vi "Tx_Create FIFO Association - Scheduled Labels - Parameters Channels.vi"(8 "error in (no error)":errorcluster, 11 "Input Channel Data []":T5[](array[typedef]) {"Labels Settings"."Label Timestamp Channel Data Reference" format="%.0x"; "Labels Settings"."Label Disable/Trigger Channel Reference" format="%.0x"; "Labels Settings"."Word"."Param Setting"."Item Refs" format="%.0x"; "Labels Settings"."Word"."Param Setting"."Num Bits" min=1 max=32; "Labels Settings"."Word"."Param Setting"."Start Bit" min=8 max=31; "Labels Settings"."Label" format="%.0o"}) -> (0 "error out":errorcluster, 2 "Raw Values":T1, 3 "Map":T4[](array[typedef]) {"Channel Data Reference" format="%.0x"})   [LabVIEW 2019, in "Ballard Arinc-429 Engine.lvlib"]
doc: "This VI creates a static association between NI-VS FIFO Channel Index and Physical Channel, Label Index, Parameter Index for Parameter Channel of a Tx Scheduled Label."
uses:
  Ballard Arinc-429 Engine.lvlib
  Shared/Controls and Global/RT HW Channel.ctl
  Shared/Controls and Global/RT Label Settings.ctl
  Shared/Controls and Global/Label.ctl
  Shared/Controls and Global/transferPeriod.ctl
  Shared/Controls and Global/RT Word Settings.ctl
  Shared/Controls and Global/RT Param Setting.ctl
  Shared/Controls and Global/Start Bit.ctl
  Shared/Controls and Global/Number of Bits.ctl
  <vilib>/NI VeriStand/Custom Device API/Block Data Reference.ctl
  <vilib>/NI VeriStand/Custom Device API/Data Reference.ctl
  <vilib>/NI VeriStand/Custom Device API/Custom Device Item Ref.ctl
  Shared/Controls and Global/TransferType.ctl
  RT Controls/RT Tx Association.ctl
  RT Controls/RT Tx Default Raw Value.ctl
  RT Controls/RT Tx Default Raw Value_Association.ctl
  <vilib>/NI VeriStand/Custom Device API/Custom Device API.lvlib
  Shared/Ballard Arinc-429 Shared.lvlib
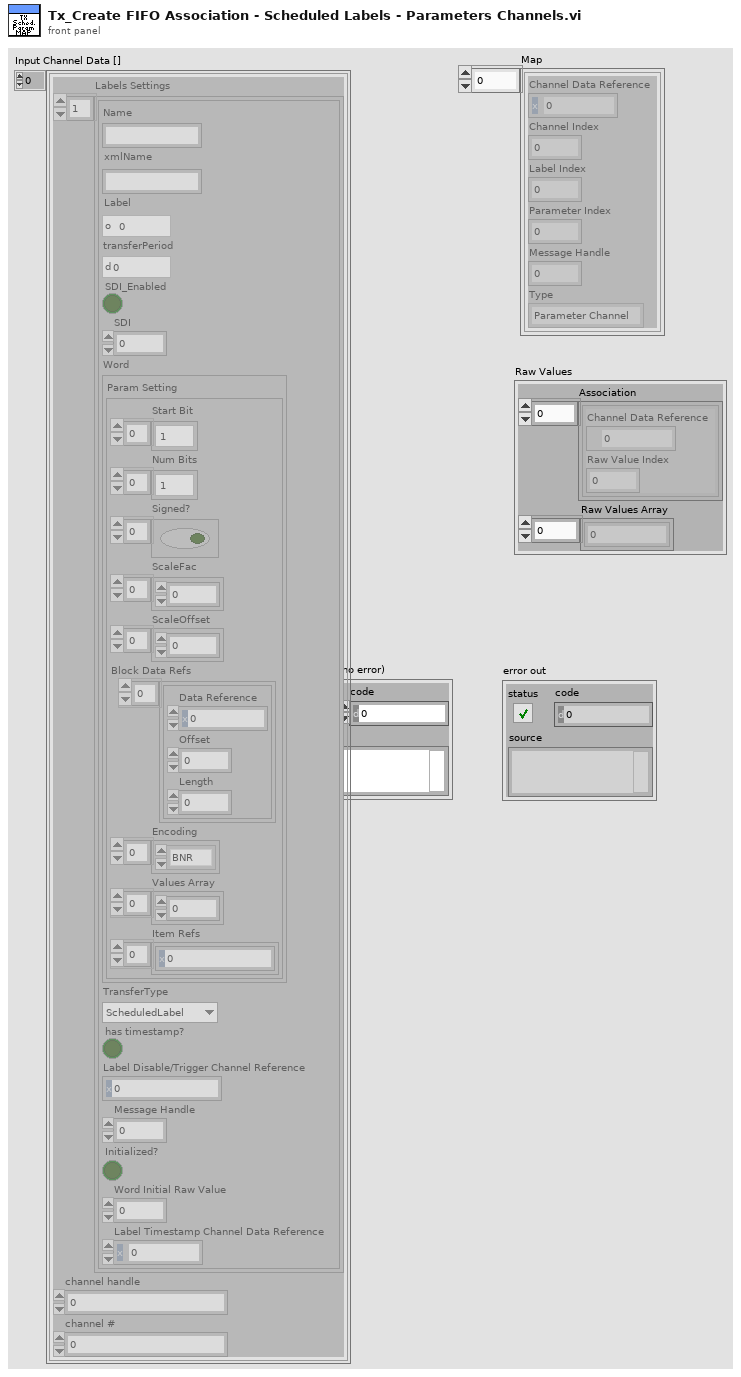
[diagram p1: front panel]
types:
  T1 = typedef "Ballard Arinc-429 Engine.lvlib/RT Tx Default Raw Value.ctl" = cluster{"Association":T2[], "Raw Values Array":u32[]}
  T2 = typedef "Ballard Arinc-429 Engine.lvlib/RT Tx Default Raw Value_Association.ctl" = cluster{"Channel Data Reference":T3, "Raw Value Index":i32}
  T3 = typedef "Custom Device API.lvlib/Data Reference.ctl" = i32
  T4 = typedef "Ballard Arinc-429 Engine.lvlib/RT Tx Association.ctl" = cluster{"Channel Data Reference":T3, "Channel Index":i32, "Label Index":i32, "Parameter Index":i32, "Message Handle":u64, "Type":enum16{"Parameter Channel", "Disable/Trigger Channel"}}
  T5 = typedef "Ballard Arinc-429 Shared.lvlib/RT HW Channel.ctl" = cluster{"Labels Settings":T6[], "channel handle":u64, "channel #":u16}
  T6 = typedef "Ballard Arinc-429 Shared.lvlib/RT Label Settings.ctl" = cluster{"Name":string, "xmlName":string, "Label":T7, "transferPeriod":T8, "SDI_Enabled":bool, "SDI":u8, "Word":T9, "TransferType":T15, "has timestamp?":bool, "Label Disable/Trigger Channel Reference":T14, "Message Handle":u64, "Initialized?":bool, "Word Initial Raw Value":u32, "Label Timestamp Channel Data Reference":T3}
  T7 = typedef "Ballard Arinc-429 Shared.lvlib/Label.ctl" = u8
  T8 = typedef "Ballard Arinc-429 Shared.lvlib/transferPeriod.ctl" = u32
  T9 = typedef "Ballard Arinc-429 Shared.lvlib/RT Word Settings.ctl" = cluster{"Param Setting":T10}
  T10 = typedef "Ballard Arinc-429 Shared.lvlib/RT Param Setting.ctl" = cluster{"Start Bit":T11[], "Num Bits":T12[], "Signed?":bool[], "ScaleFac":dbl[], "ScaleOffset":dbl[], "Block Data Refs":T13[], "Encoding":enum16{"BNR", "BCD", "Discrete"}[], "Values Array":dbl[], "Item Refs":T14[]}
  T11 = typedef "Ballard Arinc-429 Shared.lvlib/Start Bit.ctl" = i32
  T12 = typedef "Ballard Arinc-429 Shared.lvlib/Number of Bits.ctl" = i32
  T13 = typedef "Custom Device API.lvlib/Block Data Reference.ctl" = cluster{"Data Reference":T3, "Offset":u64, "Length":u64}
  T14 = typedef "Custom Device API.lvlib/Custom Device Item Ref.ctl" = u64
  T15 = typedef "Ballard Arinc-429 Shared.lvlib/TransferType.ctl" = enum16{"ScheduledLabel", "Acyclic", "Block", "Strobe"}
  T16 = enum16{"Parameter Channel", "Disable/Trigger Channel"}
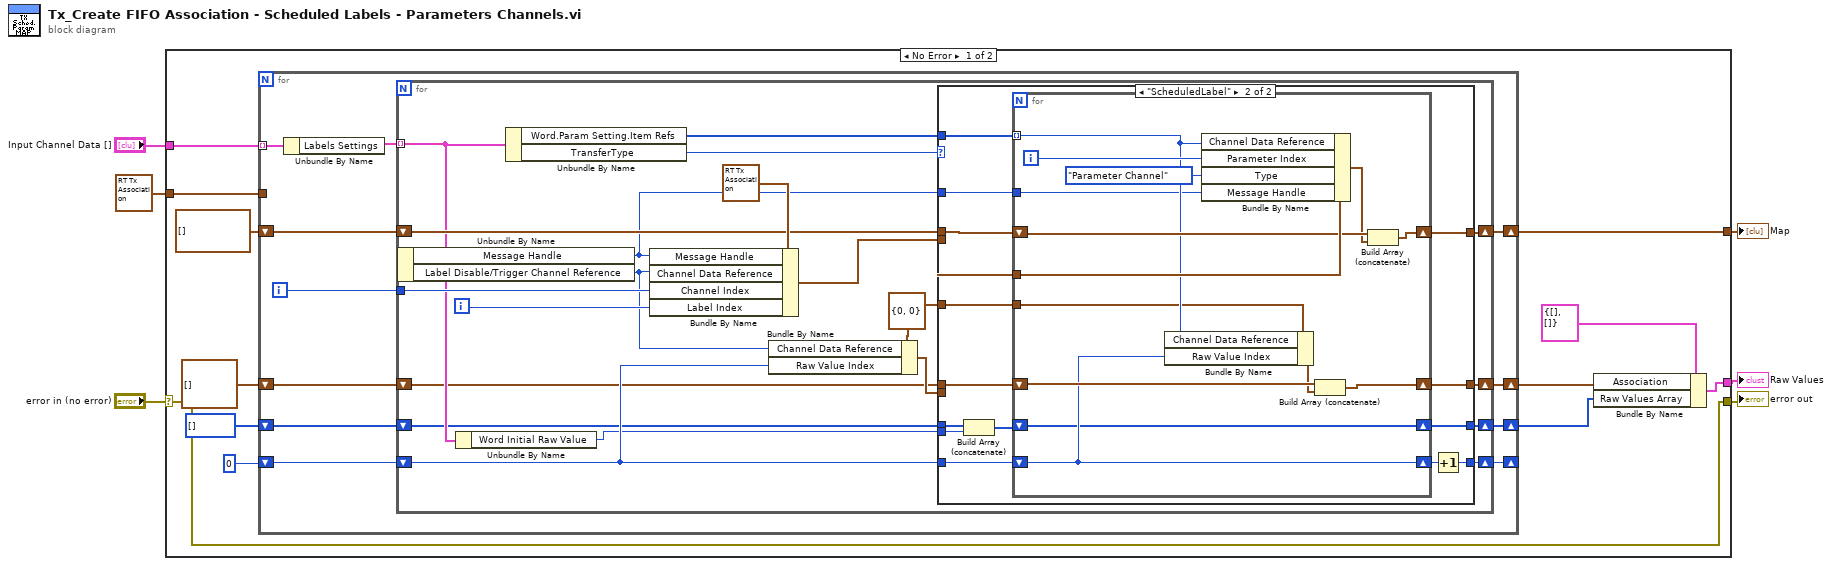
[diagram p0: block diagram]
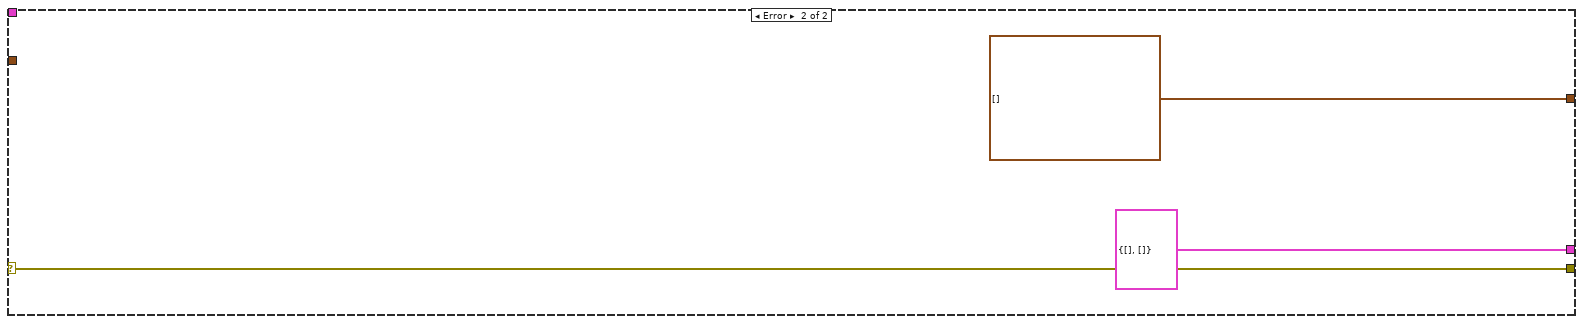
[diagram p3: hidden frame]
diagram:
  n1 = case shown="No Error" "error in (no error)" {
    selector: "error in (no error)" -> [w15 w85]
    tunnel: [w15 w85] -> w5
    tunnel: "Input Channel Data []" -> [w18 _]
    tunnel: T4 {"Channel Data Reference"=0, "Channel Index"=0, "Label Index"=0, "Parameter Index"=0, "Message Handle"=0, "Type"=enum."Parameter Channel"} ("Association") -> [w17 _]
    tunnel: [w14 T4[] []] -> w2
    tunnel: [w10 T1 {"Association"=[], "Raw Values Array"=[]}] -> w1
    frame No Error {
      n2 = for {
        tunnel: w18 -> [w28] mode=indexing
        tunnel: w17 -> [_]
        shift-right: [w25] -> w14
        shift-left: T4[] [] -> [w27]
        shift-right: [w23] -> w11
        shift-left: T2[] [] -> [w24]
        shift-right: [w19] -> w8
        shift-left: u32[] [] -> [w22]
        shift-right: [w20] -> _
        shift-left: 0 -> [w21]
        i -> [w26]
        n3 = Unbundle By Name(w28) -> ("Labels Settings"=w29:T6[])
        n4 = for {
          tunnel: w29 -> [w41] mode=indexing
          shift-right: [w46] -> w25
          shift-left: w27 -> [w47]
          tunnel: w26 -> [w48]
          shift-right: [w42] -> w23
          shift-left: w24 -> [w35]
          shift-right: [w40] -> w19
          shift-left: w22 -> [w34]
          shift-right: [w39] -> w20
          shift-left: w21 -> [w38]
          i -> [w43]
          w37 = T2 {"Channel Data Reference"=0, "Raw Value Index"=0}
          n5 = Unbundle By Name(w41) -> ("Message Handle"=w31:u64, "Label Disable/Trigger Channel Reference"=w32:T14)
          n6 = Unbundle By Name(w41) -> ("Word Initial Raw Value"=w33:u32)
          n7 = Unbundle By Name(w41) -> ("Word.Param Setting.Item Refs"=w44:T14[], "TransferType"=w30:T15)
          n8 = Bundle By Name(cluster=T4 {"Channel Data Reference"=0, "Channel Index"=0, "Label Index"=0, "Parameter Index"=-1, "Message Handle"=0, "Type"=enum."Disable/Trigger Channel"} ("Association"), "Message Handle"=w31, "Channel Data Reference"=w32, "Channel Index"=w48, "Label Index"=w43) -> (w45:T4)
          n9 = Bundle By Name(cluster=w37, "Channel Data Reference"=w32, "Raw Value Index"=w38) -> (w36:T2)
          n10 = case shown="\"ScheduledLabel\"" w30 {
            tunnel: w47 -> [w53 w68]
            tunnel: [w53 w67] -> w46
            tunnel: w45 -> [_ w66]
            tunnel: w44 -> [_ w65]
            tunnel: [w52 w64] -> w42
            tunnel: [w51 w63] -> w40
            tunnel: [w50 w61] -> w39
            tunnel: w38 -> [w50 w60]
            tunnel: w37 -> [_ w59]
            tunnel: w36 -> [_ _]
            tunnel: w35 -> [w52 w58]
            tunnel: w34 -> [w51 w57]
            tunnel: w33 -> [_ w56]
            tunnel: w31 -> [_ w54]
            frame Default {
            }
            frame "ScheduledLabel" {
              n11 = Build Array (concatenate)(w57, w56) -> (w55:u32[])
              n12 = for {
                shift-right: [w79] -> w67
                shift-left: w68 -> [w81]
                tunnel: w66 -> [w82]
                tunnel: w65 -> [w74] mode=indexing
                shift-right: [w76] -> w64
                shift-left: w58 -> [w77]
                shift-right: [w71] -> w63
                shift-left: w55 -> [w71]
                shift-right: [w75] -> w62
                shift-left: w60 -> [w75]
                tunnel: w59 -> [w72]
                tunnel: w54 -> [w70]
                i -> [w78]
                n13 = Bundle By Name(cluster=w72, "Channel Data Reference"=w74, "Raw Value Index"=w75) -> (w73:T2)
                n14 = Bundle By Name(cluster=w82, "Channel Data Reference"=w74, "Parameter Index"=w78, "Type"=T16."Parameter Channel", "Message Handle"=w70) -> (w80:T4)
                n15 = Build Array (concatenate)(w77, w73) -> (w76:T2[])
                n16 = Build Array (concatenate)(w81, w80) -> (w79:T4[])
              }
              n17 = Increment(x=w62) -> (x+1=w61:i32)
            }
          }
        }
      }
      n18 = Bundle By Name(cluster=T1 {"Association"=[], "Raw Values Array"=[]} ("Raw Values"), "Association"=w11, "Raw Values Array"=w8) -> (w10:T1)
    }
    frame Error {
    }
  }
  "error out" <- w5
  "Map" <- w2
  "Raw Values" <- w1
